vi "Test.vi"() -> ()   [LabVIEW 2013]
panel:
  in  "불리언":bool
  in  "숫자형":dbl
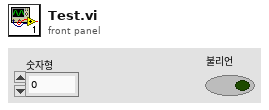
[diagram p1: front panel]
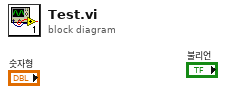
[diagram p0: block diagram]
diagram:
